vi "Actor Core.vi"(8 "error in":errorcluster, 11 "CS++GUIActor in":refnum<class "CS++GUIActor.lvclass">) -> (0 "error out":errorcluster, 3 "Actor out":refnum<class "Actor.lvclass">)   [LabVIEW 2014, in "CS++GUIActor.lvlib" / "CS++GUIActor.lvclass"]
doc: "(<B>Filename</B>: Actor Framework.lvlib:Actor.lvclass:Actor Core.vi)\n\nReceives messages to the actor, reacts to them, and initiates any error handling that may shut the actor down.\n\nDescendant classes may override this VI to append parallel tasks for the actor to complete while it handles messages. Overrides use the Call Parent Method node."
uses:
  CS++GUIActor.lvclass
  <vilib>/ActorFramework/Actor/Actor.lvclass
  CS++BaseActor/CS++BaseActor.lvclass/CS++BaseActor.ctl
  CS++GUIActor.lvclass/CS++GUIActor.ctl
  <vilib>/ActorFramework/Actor/Actor.lvclass/Actor.ctl
  <vilib>/ActorFramework/Message Enqueuer/Message Enqueuer.lvclass/Message Enqueuer.ctl
  CS++BaseActor/Read Object Name.vi
  Read Associated Actor Name.vi
  Read Stop-Event.vi
  Read PV-Update.vi
  <vilib>/ActorFramework/Message Enqueuer/Enqueue.vi
  <vilib>/ActorFramework/Message Enqueuer/Init from Existing Queue.vi
  <vilib>/ActorFramework/Message Priority Queue/Priority Enqueue.vi
  <vilib>/ActorFramework/Stop Msg/Stop Msg.lvclass
  <vilib>/ActorFramework/Message Enqueuer/Message Enqueuer.lvclass
  Classes/CS++ProcessVariables/ProcessVariable/PV.lvclass
  CS++BaseActor/CS++BaseActor.lvclass
  Libraries/Utilities/CS++Utilities.lvlib
panel:
  in  "Stop Button":bool
  out "Associated DeviceActor":string
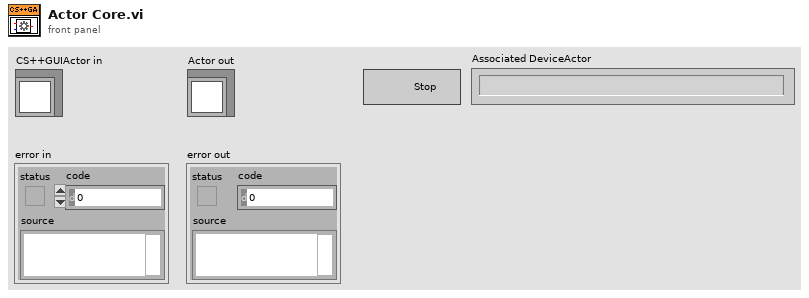
[diagram p1: front panel]
types:
  T1 = enum32{"Invalid", "Standard", "Closed", "Hidden", "Minimized", "Maximized"}
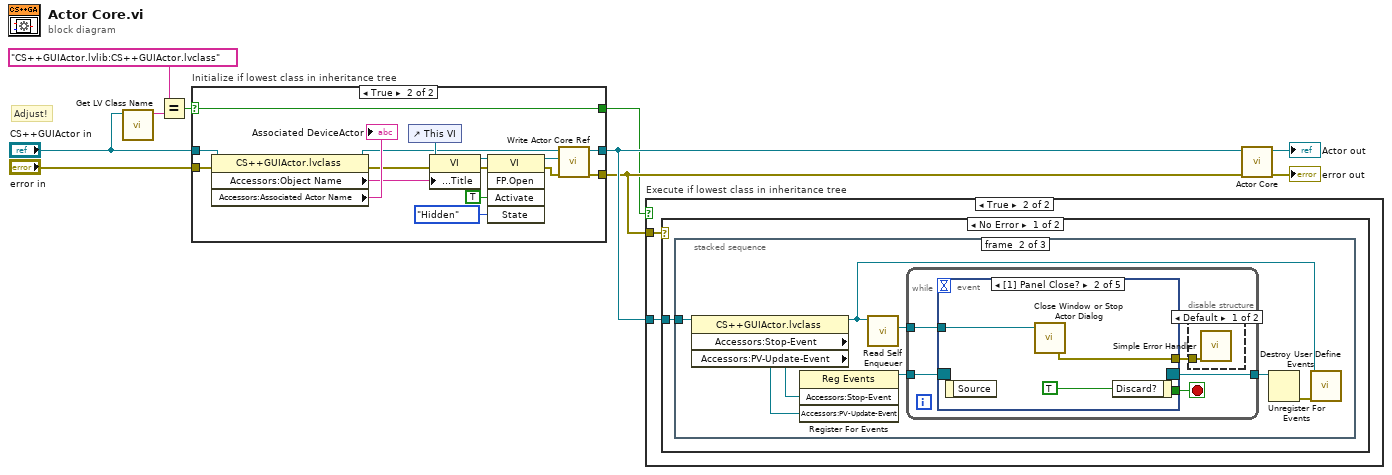
[diagram p0: block diagram]
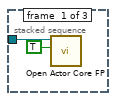
[diagram p3: hidden frame]
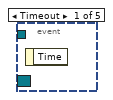
[diagram p5: hidden frame]
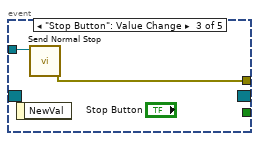
[diagram p6: hidden frame]
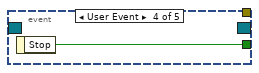
[diagram p7: hidden frame]
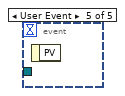
[diagram p8: hidden frame]
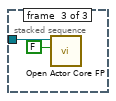
[diagram p9: hidden frame]
diagram:
  # "Adjust!"
  n1 = call <vilib>:"Get LV Class Name.vi"("object"="CS++GUIActor in") -> ("class name"=w9:string)  [unwired: 9 in, 1 out]
  n2 = Equal?(x="CS++GUIActor.lvlib:CS++GUIActor.lvclass" ("class name"), y=w9) -> (x = y?=w2:bool)
  n3 = case "Initialize if lowest class in inheritance tree" shown="True" w2 {
    selector: w2 -> [w13 w27]
    tunnel: "error in" -> [w11 w24]
    tunnel: "CS++GUIActor in" -> [w12 w25]
    tunnel: [w12 w21] -> w4
    tunnel: [w11 w20] -> w3
    tunnel: [w13 w27] -> w1
    frame False {
    }
    frame True {
      n4 = property class="CS++GUIActor.lvclass"(reference=w25, error in=w24) -> (reference out=w14:refnum<class "CS++GUIActor.lvclass">, error out=w16:errorcluster, "Accessors:Object Name"=w15:string, "Accessors:Associated Actor Name"=→"Associated DeviceActor":string)
      n5 = control-ref of="This VI"() -> (w19:refnum<vi>)
      n6 = property class="VI"(reference=w19, error in=w16, "Front Panel.Title"=w15) -> (reference out=w18:refnum<vi>, error out=w17:errorcluster)
      n7 = invoke class="VI" method="FP.Open"(reference=w18, error in=w17, "Activate"=TRUE ("Activate?"), "State"=T1."Hidden") -> (reference out=w26:refnum<vi>, error out=w22:errorcluster)  [unwired: 1 in, 3 out]
      n8 = call "Write Actor Core Ref.vi"("error in (no error)"=w22, "Actor Core Ref"=w26, "CS++BaseActor in"=w14) -> ("error out"=w20:errorcluster, "CS++BaseActor out"=w21:refnum<class "CS++GUIActor.lvclass">)  [unwired: 7 in]
    }
  }
  n9 = case "Execute if lowest class in inheritance tree" shown="True" w1 {
    tunnel: w4 -> [_ w31]
    tunnel: w3 -> [_ w30]
    frame False {
    }
    frame True {
      n10 = case shown="No Error" w30 {
        tunnel: w31 -> [w32 _]
        frame No Error {
          n11 = stacked-sequence {
            tunnel: w32 -> [w34 w42 w56]
            frame #0 {
              n12 = call "Open Actor Core FP.vi"("Open FP (F)"=TRUE, "CS++BaseActor in"=w34) -> ()  [unwired: 8 in, 2 out]
            }
            frame #1 {
              n13 = property class="CS++GUIActor.lvclass"(reference=w42) -> (reference out=w39:refnum<class "CS++GUIActor.lvclass">, "Accessors:Stop-Event"=w36:refnum<user-event>, "Accessors:PV-Update-Event"=w35:refnum<user-event>)  [unwired: 1 in, 1 out]
              n14 = register-events(w36, w35) -> (reference out=w37:refnum<event-registration>)  [unwired: 2 in, 1 out]
              n15 = call <vilib>:"Read Self Enqueuer.vi"("Actor"=w39) -> ("Self Enqueuer"=w38:refnum<class "Message Enqueuer.lvclass">)  [unwired: 10 in]
              n16 = while {
                tunnel: w37 -> [w47]
                tunnel: [w45] -> w41
                tunnel: w38 -> [w43]
                stop <- w46 stop-if-true
                n17 = event shown="[1] Panel Close?" {
                  selector: w47 -> [_ _ _ _ _]
                  dyn-events: [_ _ _ _ _] -> w45
                  timeout: _ -> [_ _ _ _ _]
                  tunnel: [_ _ _ w54 _] -> w46
                  tunnel: [_ w49 w53 _ _] -> w44
                  tunnel: w43 -> [_ w50 w52 _ _]
                  event Timeout {
                    n18 = event-data() -> ()  [unwired: 1 in, 1 out]
                  }
                  event Panel Close? {
                    n19 = event-data() -> ()  [unwired: 1 in, 1 out]
                    n20 = call "Close Window or Stop Actor Dialog.vi"("Self Enqueuer"=w50) -> ("Error Out"=w49:errorcluster)  [unwired: 2 in]
                    n21 = event-data("Discard?"=TRUE) -> ()  [unwired: 1 in, 1 out]
                  }
                  event "Stop Button": Value Change {
                    n22 = event-data() -> ()  [unwired: 1 in, 1 out]
                    n23 = call <vilib>:"Send Normal Stop.vi"("Message Enqueuer"=w52) -> ("error out"=w53:errorcluster)  [unwired: 10 in]
                  }
                  event User Event {
                    n24 = event-data() -> ("Stop"=w54:bool)  [unwired: 1 in]
                  }
                  event User Event {
                    n25 = event-data() -> ()  [unwired: 1 in, 1 out]
                  }
                }
                n26 = disable-structure shown="Default" {
                  disable-tunnel: w44 -> [w48 _]
                  frame condition #0 (active) {
                    n27 = call <vilib>:"Simple Error Handler.vi"("error in (no error)"=w48) -> ()  [unwired: 4 in, 5 out]
                  }
                  frame condition #1 {
                  }
                }
              }
              n28 = Unregister For Events(event registration refnum=w41) -> (error out=w40:errorcluster)  [unwired: 1 in]
              n29 = call-dynamic "Destroy User Define Events.vi"("error in (no error)"=w40, "CS++GUIActor in"=w39) -> ()  [unwired: 8 in, 2 out]
            }
            frame #2 {
              n30 = call "Open Actor Core FP.vi"("Open FP (F)"=FALSE, "CS++BaseActor in"=w56) -> ()  [unwired: 8 in, 2 out]
            }
          }
        }
        frame Error {
        }
      }
    }
  }
  n31 = call-parent "Actor Core.vi"("error in"=w3, "CS++BaseActor in"=w4) -> ("error out"=→"error out":errorcluster, "Actor out"=→"Actor out":refnum<class "Actor.lvclass">)  [unwired: 8 in]
